vi "update_modifier_signals.vi"(8 "error in (no error)":errorcluster, 11 "DL090202ScanHead in":refnum<class "ScanHeadDL090202.lvclass">) -> (0 "error out":errorcluster, 3 "DL090202ScanHead out":refnum<class "ScanHeadDL090202.lvclass">)   [LabVIEW 2010]
uses:
  GenericScanHead/GenericScanHead/GenericScanHead.lvclass
  Trajectory/GenericTrajectory/GenericTrajectory/GenericTrajectory.lvclass
  ScanHeadDL090202.lvclass
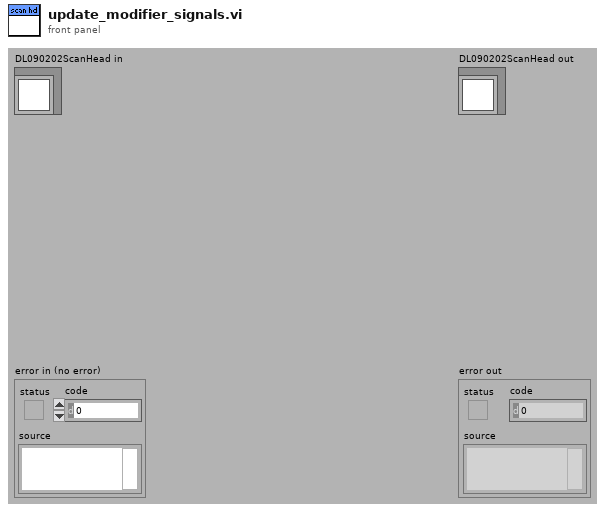
[diagram p1: front panel]
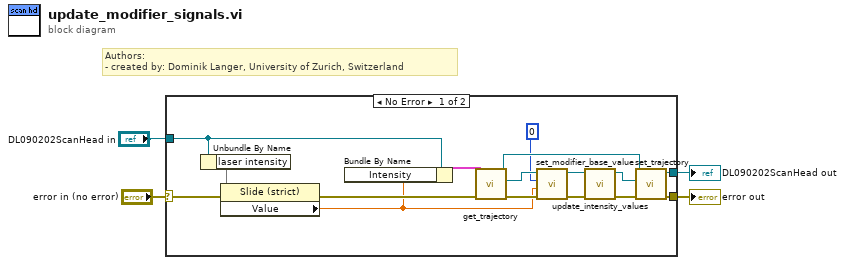
[diagram p0: block diagram]
diagram:
  # "Authors: \n- created by: Dominik Langer, University of Zurich, Switzerland"
  n1 = case shown="No Error" "error in (no error)" {
    selector: "error in (no error)" -> [w10 w22]
    tunnel: [w19 w22] -> w3
    tunnel: [w20 w21] -> w1
    tunnel: "DL090202ScanHead in" -> [w7 w21]
    frame No Error {
      n2 = Unbundle By Name(w7) -> ("laser intensity"=w8)
      n3 = property class="Slide (strict)"(reference=w8, error in=w10) -> (error out=w9:errorcluster, "Value"=w5:dbl)  [unwired: 1 out]
      n4 = Bundle By Name(cluster=w7, "Intensity"=w5) -> (w6:cluster{})
      n5 = call-dynamic "get_trajectory.vi"("error in (no error)"=w9, "GenericScanHead.lvclass in"=w6) -> ("error out"=w16:errorcluster, "trajectory"=w17:refnum<class "GenericTrajectory.lvclass">, "GenericScanHead.lvclass out"=w18:refnum<class "GenericScanHead.lvclass">)  [unwired: 7 out]
      n6 = call-dynamic "set_modifier_base_value.vi"("error in (no error)"=w16, "modifier base value"=w5, "modifier index"=0, "GenericTrajectory.lvclass in"=w17) -> ("error out"=w14:errorcluster, "GenericTrajectory.lvclass out"=w13:refnum<class "GenericTrajectory.lvclass">)  [unwired: 6 out]
      n7 = call-dynamic "update_intensity_values.vi"("error in (no error)"=w14, "GenericTrajectory in"=w13) -> ("error out"=w12:errorcluster, "GenericTrajectory out"=w11:refnum<class "GenericTrajectory.lvclass">)  [unwired: 8 out]
      n8 = call-dynamic "set_trajectory.vi"("error in (no error)"=w12, "trajectory"=w11, "GenericScanHead.lvclass in"=w18) -> ("error out"=w19:errorcluster, "GenericScanHead.lvclass out"=w20:refnum<class "GenericScanHead.lvclass">)  [unwired: 7 out]
    }
    frame Error {
    }
  }
  "error out" <- w3
  "DL090202ScanHead out" <- w1
